vi "Send Start Streaming.vi"(7 "Message Priority (Normal)":T2=enum."Normal", 8 "error in (no error)":errorcluster, 10 "Camera Settings":T1={"Exposure Time (ms)"=100.0, "Binning"=enum."2x2", "Scan Mode"=-1, "Frames to Acquire"=1000.0, "Pixel Correction"=FALSE, "Frames to Skip"=1, "File Path"=path "", "Duty cycle"=1.0, "ALEX"=FALSE, "Shutter Enable"=[], "fluidics trigger frame"=0, "Bit Depth"=16, "Image Width (px)"=0, "Image Height (px)"=0, "Horizontal Offset (px)"=0, "Vertical Offset (px)"=0} {"fluidics trigger frame" max=60000 step=1; "Exposure Time (ms)" min=1.0 max=10000.0 step=1.0}, 11 "Message Enqueuer":refnum<class "Message Enqueuer.lvclass">) -> (0 "error out":errorcluster, 3 "Message Enqueuer out":refnum<class "Message Enqueuer.lvclass">)   [LabVIEW 2023, in "Sync Device.lvlib" / "Start Streaming Msg.lvclass"]
doc: "This VI sends the message to an actor."
uses:
  Start Streaming Msg.lvclass
  <vilib>/ActorFramework/Message Enqueuer/Message Enqueuer.lvclass
  <vilib>/ActorFramework/Message Enqueuer/Message Priority.ctl
  Resources/Type Defs/Camera Settings.ctl
  C:/Program Files/National Instruments/LabVIEW 2023/vi.lib/ActorFramework/Message/Message.lvclass
  Start Streaming Msg.lvclass/Start Streaming Msg.ctl
  <vilib>/ActorFramework/Message Enqueuer/Message Enqueuer.lvclass/Message Enqueuer.ctl
  <vilib>/ActorFramework/Message Priority Queue/Priority Enqueue.vi
  C:/FlashGordon/Development/Hardware/Sync Device Messages/Start Streaming Msg/Start Streaming Msg.lvclass
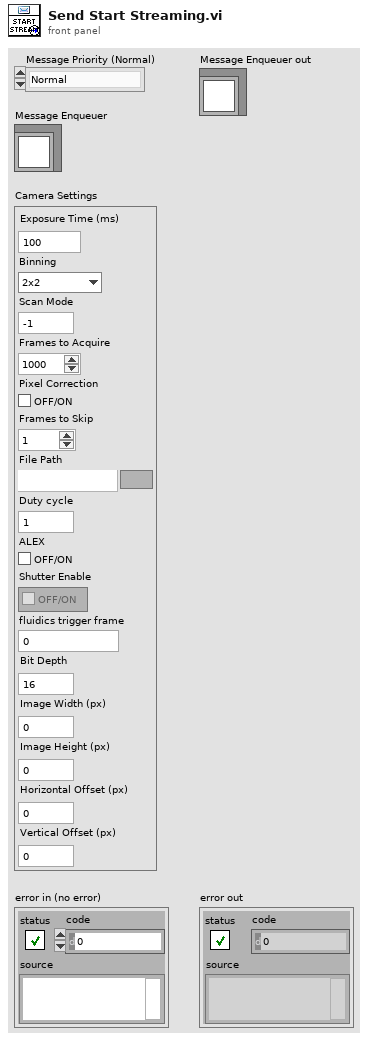
[diagram p1: front panel]
types:
  T1 = typedef "Camera Settings.ctl" = cluster{"Exposure Time (ms)":dbl, "Binning":enum16{"1x1", "2x2", "4x4"}, "Scan Mode":i32, "Frames to Acquire":dbl, "Pixel Correction":bool, "Frames to Skip":u32, "File Path":path, "Duty cycle":dbl, "ALEX":bool, "Shutter Enable":bool[], "fluidics trigger frame":u16, "Bit Depth":u16, "Image Width (px)":u16, "Image Height (px)":u16, "Horizontal Offset (px)":u16, "Vertical Offset (px)":u16}
  T2 = typedef "Actor Framework.lvlib/Message Enqueuer.lvclass/Message Priority.ctl" = enum16{"Low", "Normal", "High"}
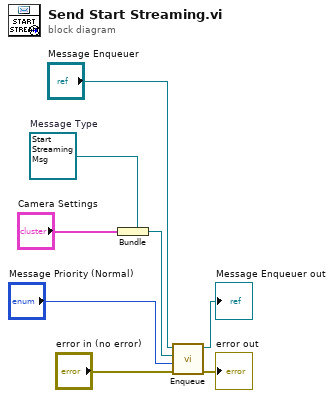
[diagram p0: block diagram]
diagram:
  w5 = refnum<class "Start Streaming Msg.lvclass"> refnum  # Message Type
  n1 = Bundle(cluster=w5, "Camera Settings") -> (w4:refnum<class "Start Streaming Msg.lvclass">)
  n2 = call <vilib>:"Enqueue.vi"("error in (no error)"="error in (no error)", "Message Priority (Normal)"="Message Priority (Normal)", "Message"=w4, "Message Enqueuer in"="Message Enqueuer") -> ("error out"=→"error out":errorcluster, "Message Enqueuer in"=→"Message Enqueuer out":refnum<class "Message Enqueuer.lvclass">)  [unwired: 6 in]
